vi "LockInQueues_GET.vi"(8 "error in":errorcluster, 11 "lia host in":refnum<class "LIA Host Interface RT.lvclass">) -> (0 "error out":errorcluster, 2 "lock-in queues":refnum<queue>[](array[refnum]), 3 "lia host out":refnum<class "LIA Host Interface RT.lvclass">)   [LabVIEW 2018, in "LIA Host Interface RT.lvclass"]
uses:
  LIA Host Interface RT.lvclass
  LIA Host Interface RT.lvclass/LIA Host Interface RT.ctl
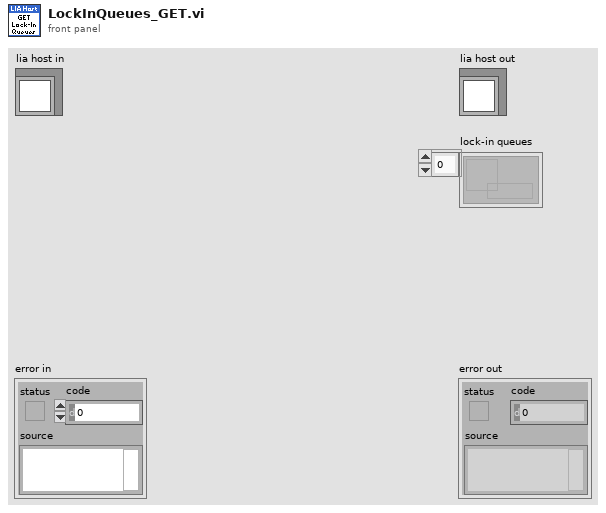
[diagram p1: front panel]
types:
  T1 = typedef "Lock-In Amplifier Host RT.lvclass/session data.ctl" = cluster{"tcp connection":refnum<k5>, "incoming data":refnum<queue>, "outgoing data":refnum<queue>, "lock-in data":refnum<queue>[], "stop process":refnum<notifier>}
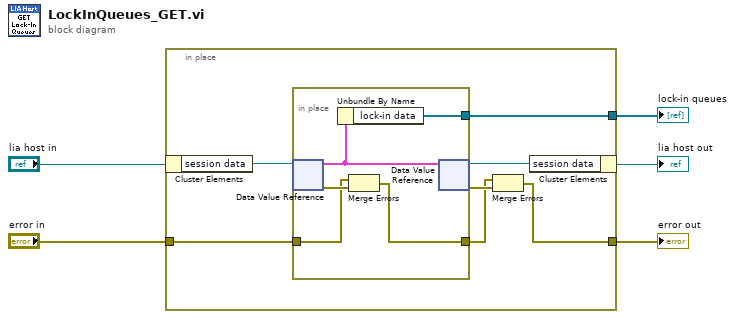
[diagram p0: block diagram]
diagram:
  n1 = in-place {
    in-place-border: [w10] -> w1
    in-place-border: "error in" -> [w9]
    in-place-border: [w6] -> w2
    n2 = in-place-cluster #1("lia host in") -> ("session data"=w12:refnum<data-value>)
    n3 = in-place {
      in-place-border: [w16] -> w10
      in-place-border: w9 -> [w14]
      in-place-border: [w13] -> w7
      n4 = in-place-dvr #2(w12) -> (w17:T1, w15:errorcluster)
      n5 = Unbundle By Name(w17) -> ("lock-in data"=w16:refnum<queue>[])
      n6 = Merge Errors(w14, w15) -> (w13:errorcluster)
      n7 = in-place-dvr #2(w17) -> (w11:refnum<data-value>, w8:errorcluster)
    }
    n8 = Merge Errors(w7, w8) -> (w6:errorcluster)
    n9 = in-place-cluster #1("session data"=w11) -> (→"lia host out":refnum<class "LIA Host Interface RT.lvclass">)
  }
  "error out" <- w2
  "lock-in queues" <- w1
